vi "ma_Tone estimation subroutine G(f) (first derivative, FFT input).vi"(1 "N (window length)":i32=512, 2 "window":u16(ring) items=["Rectangle"=0, "Hanning"=1, "Hamming"=2, "Blackman-Harris"=3, "Exact Blackman"=4, "Blackman"=5, "Flat Top"=6, "4 Term B-Harris "=7, "7 Term B-Harris"=8, "Low Sidelobe"=9, "Blackman Nuttall"=11, "Triangle"=30, "Bartlett-Hanning"=31, "Bohman"=32, "Parzen"=33, "Welch"=34, "Kaiser"=60, "Dolph-Chebyshev"=61, "Gaussian"=62], 3 "frequency":dbl format="%.5f", 4 "three fingers":T1={"f0"=0.0, "df"=1.0, "spectrum"=[]} {"spectrum" format="%.2f"; "df" format="%.2f"; "f0" format="%.2f"}) -> (0 "G'(f)":dbl format="%.2f")   [LabVIEW 2020, in "NI_MAPro.lvlib"]
uses:
  NI_MAPro.lvlib
  ma_sml_Spectrum Cluster (complex).ctl
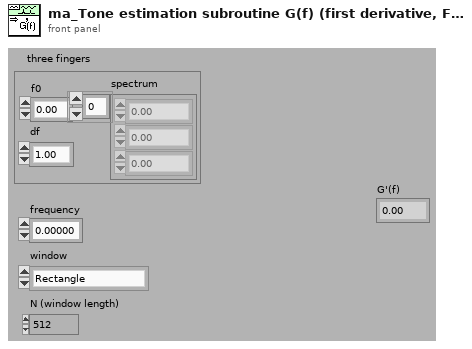
[diagram p1: front panel]
types:
  T1 = typedef "NI_MAPro.lvlib/ma_sml_Spectrum Cluster (complex).ctl" = cluster{"f0":dbl, "df":dbl, "spectrum":cdb[]}
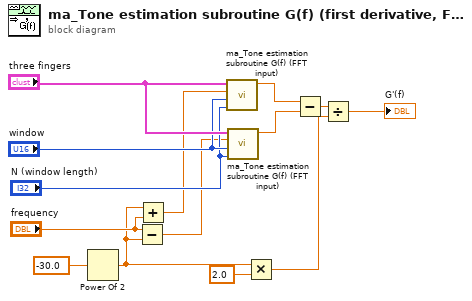
[diagram p0: block diagram]
diagram:
  n1 = Power Of 2(x=-30.0) -> (2^x=w3:dbl)
  n2 = Subtract(x="frequency", y=w3) -> (x-y=w4:dbl)
  n3 = Add(x=w3, y="frequency") -> (x+y=w9:dbl)
  n4 = call "ma_Tone estimation subroutine G(f) (FFT input).vi"("N (window length)"="N (window length)", "window"="window", "frequency"=w9, "three fingers"="three fingers") -> ("G(f)"=w8:dbl)  [unwired: 1 in, 2 out]
  n5 = call "ma_Tone estimation subroutine G(f) (FFT input).vi"("N (window length)"="N (window length)", "window"="window", "frequency"=w4, "three fingers"="three fingers") -> ("G(f)"=w7:dbl)  [unwired: 1 in, 2 out]
  n6 = Multiply(x=w3, y=2.0) -> (x*y=w2:dbl)
  n7 = Subtract(x=w8, y=w7) -> (x-y=w6:dbl)
  n8 = Divide(x=w6, y=w2) -> (x/y=→"G'(f)":dbl)
